vi "SVM Train ONE_CLASS.vi"(7 "Options":T2={"cache_size"=200.0, "eps"=0.001, "shrinking"=TRUE, "probability"=FALSE}, 8 "error in (no error)":errorcluster, 9 "nu":T1=0.5 caption="nu (0,5)", 10 "Kernel":T9, 11 "Problem":T8) -> (0 "error out":errorcluster, 3 "Model":T3)   [LabVIEW 2015]
doc: "This function constructs and returns an SVM model according to the given training data and parameters."
uses:
  Controls/Kernel.ctl
  Wrapper API/Controls/svm_kernel_type.ctl
  Wrapper API/Controls/svm_problem.ctl
  Wrapper API/Controls/svm_node.ctl
  Wrapper API/Controls/svm_model.ctl
  Wrapper API/Controls/svm_parameter.ctl
  Wrapper API/Controls/svm_type.ctl
  Controls/Options Training.ctl
  Controls/Parameters ONE_CLASS.ctl
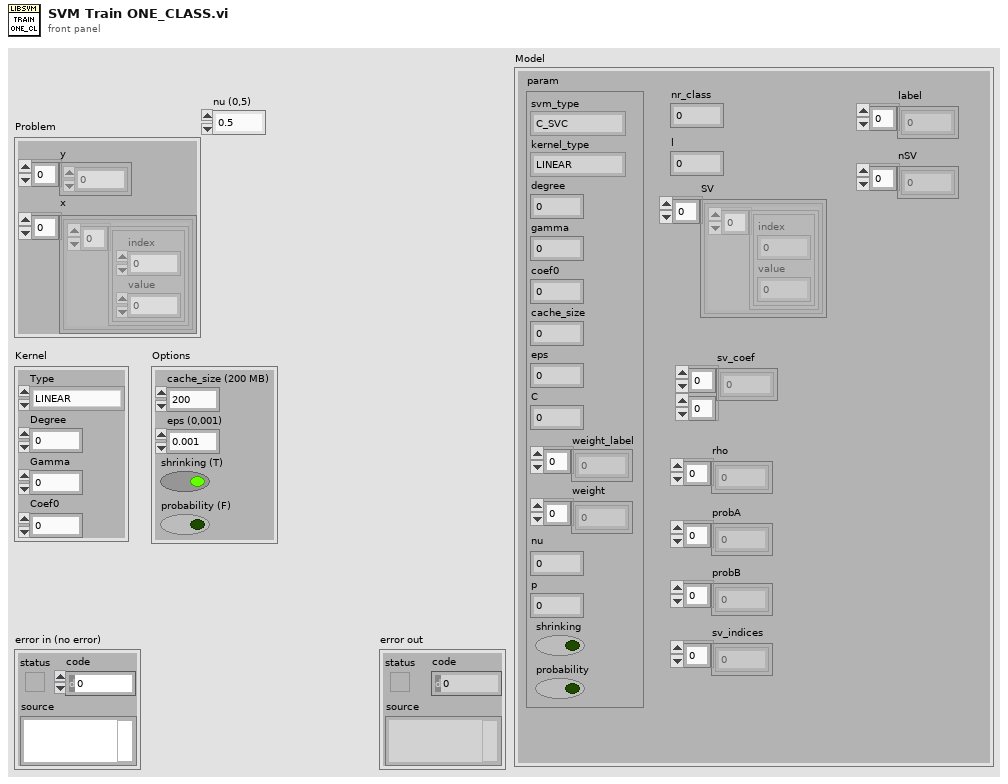
[diagram p1: front panel]
types:
  T1 = typedef "Parameters ONE_CLASS.ctl" = dbl
  T2 = typedef "Options Training.ctl" = cluster{"cache_size":dbl, "eps":dbl, "shrinking":bool, "probability":bool}
  T3 = typedef "svm_model.ctl" = cluster{"param":T4, "nr_class":i32, "l":i32, "SV":cluster{"Array":T7[]}[], "sv_coef":dbl[][], "rho":dbl[], "probA":dbl[], "probB":dbl[], "sv_indices":i32[], "label":i32[], "nSV":i32[]}
  T4 = typedef "svm_parameter.ctl" = cluster{"svm_type":T5, "kernel_type":T6, "degree":i32, "gamma":dbl, "coef0":dbl, "cache_size":dbl, "eps":dbl, "C":dbl, "weight_label":i32[], "weight":dbl[], "nu":dbl, "p":dbl, "shrinking":bool, "probability":bool}
  T5 = typedef "svm_type.ctl" = enum32{"C_SVC", "NU_SVC", "ONE_CLASS", "EPSILON_SVR", "NU_SVR"}
  T6 = typedef "svm_kernel_type.ctl" = enum32{"LINEAR", "POLY", "RBF", "SIGMOID", "PRECOMPUTED"}
  T7 = typedef "svm_node.ctl" = cluster{"index":i32, "value":dbl}
  T8 = typedef "svm_problem.ctl" = cluster{"y":dbl[], "x":cluster{T7[]}[]}
  T9 = typedef "Kernel.ctl" = cluster{"Type":T6, "Degree":i32, "Gamma":dbl, "Coef0":dbl}
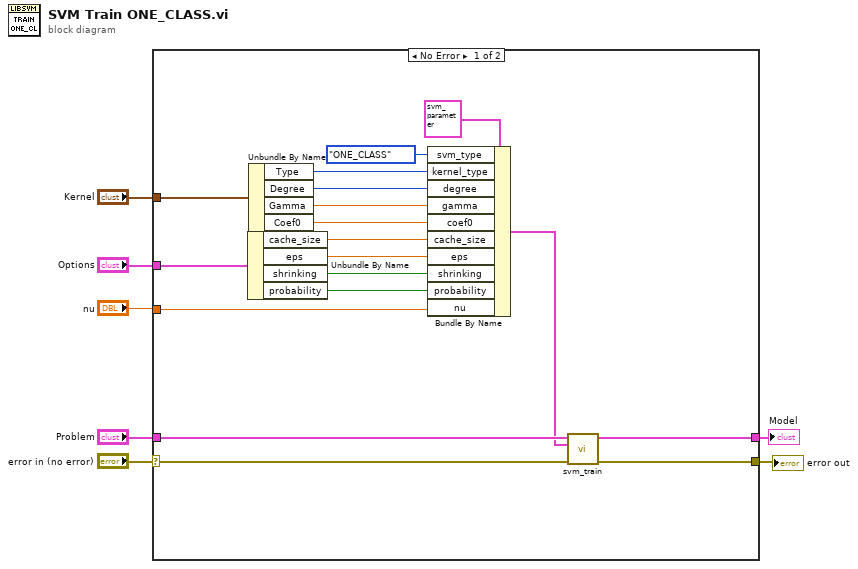
[diagram p0: block diagram]
diagram:
  n1 = case shown="No Error" "error in (no error)" {
    selector: "error in (no error)" -> [w25 w26]
    tunnel: [w24 w26] -> w7
    tunnel: "Problem" -> [w22 _]
    tunnel: "Kernel" -> [w21 _]
    tunnel: [w14 _] -> w3
    tunnel: "Options" -> [w11 _]
    tunnel: "nu" -> [w8 _]
    frame No Error {
      n2 = Unbundle By Name(w11) -> ("cache_size"=w13:dbl, "eps"=w12:dbl, "shrinking"=w10:bool, "probability"=w9:bool)
      n3 = Unbundle By Name(w21) -> ("Type"=w20:T6, "Degree"=w19:i32, "Gamma"=w18:dbl, "Coef0"=w17:dbl)
      n4 = Bundle By Name(cluster=T4 {"svm_type"=enum."C_SVC", "kernel_type"=enum."LINEAR", "degree"=0, "gamma"=0.0, "coef0"=0.0, "cache_size"=0.0, "eps"=0.0, "C"=0.0, "weight_label"=[], "weight"=[], "nu"=0.0, "p"=0.0, "shrinking"=FALSE, "probability"=FALSE} ("svm_parameter"), "svm_type"=svm_type."ONE_CLASS", "kernel_type"=w20, "degree"=w19, "gamma"=w18, "coef0"=w17, "cache_size"=w13, "eps"=w12, "shrinking"=w10, "probability"=w9, "nu"=w8) -> (w15:T4)
      n5 = call "svm_train.vi"("error in (no error)"=w25, "Parameters"=w15, "Problem"=w22) -> ("error out"=w24:errorcluster, "Model"=w14:T3)  [unwired: 7 in]
    }
    frame Error {
    }
  }
  "error out" <- w7
  "Model" <- w3
